vi "Send MoveBySteps.vi"(5 "Polarity":enum16{"Positive", "Negative"}(ring), 6 "Direction":enum16{"Forward", "Backwards"}(ring), 7 "Message Priority (Normal)":T1=enum."Normal", 8 "error in (no error)":errorcluster, 9 "Speed":u32, 10 "Steps":u32, 11 "Message Enqueuer":refnum<class "Message Enqueuer.lvclass">) -> (0 "error out":errorcluster, 3 "Message Enqueuer out":refnum<class "Message Enqueuer.lvclass">)   [LabVIEW 2023, in "ArduinoTranslationStage.lvlib" / "MoveBySteps Msg.lvclass"]
doc: "This VI sends the message to an actor."
uses:
  MoveBySteps Msg.lvclass
  <vilib>/ActorFramework/Message Enqueuer/Message Enqueuer.lvclass
  <vilib>/ActorFramework/Message Enqueuer/Message Priority.ctl
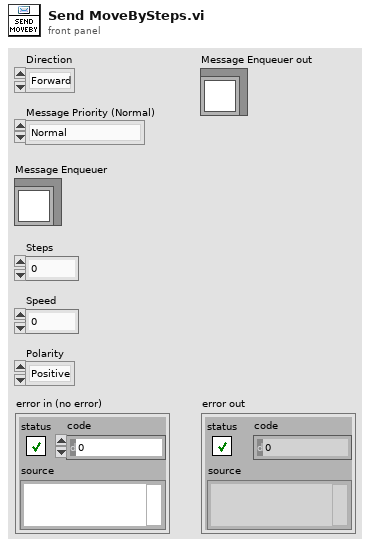
[diagram p1: front panel]
types:
  T1 = typedef "Actor Framework.lvlib/Message Enqueuer.lvclass/Message Priority.ctl" = enum16{"Low", "Normal", "High"}
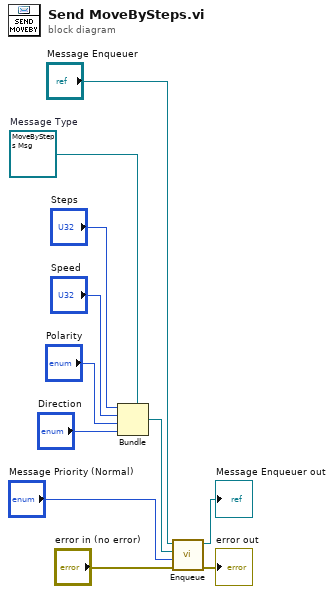
[diagram p0: block diagram]
diagram:
  w8 = refnum<class "MoveBySteps Msg.lvclass"> refnum  # Message Type
  n1 = Bundle(cluster=w8, "Steps", "Speed", "Polarity", "Direction") -> (w7:refnum<class "MoveBySteps Msg.lvclass">)
  n2 = call <vilib>:"Enqueue.vi"("error in (no error)"="error in (no error)", "Message Priority (Normal)"="Message Priority (Normal)", "Message"=w7, "Message Enqueuer in"="Message Enqueuer") -> ("error out"=→"error out":errorcluster, "Message Enqueuer out"=→"Message Enqueuer out":refnum<class "Message Enqueuer.lvclass">)  [unwired: 6 in]
